vi "IV.vi"(2 "Run uninterrupted?":bool, 3 "Device Category IN:":string(combo)="R0" caption="Device Category:", 4 "Batch No.:":string, 5 "Wafer Serial No.:":string, 6 "Sensor Serial No.:":string) -> (0 "Done!":bool)   [LabVIEW 2018]
doc: "Performs IV measurements according to ATLAS ITk Quality Control Specifications."
uses:
  general_VIs/globals/QC_MeasurementSetup.vi
  general_VIs/globals/QC_RunInformation.vi
  InstrControl/InstrumentSetup.vi
  InstrControl/Switching/Switching.lvclass
  InstrControl/SupplyControl/SupplyControl.lvclass
  InstrControl/ArduinoControl/ArduinoControl.lvclass
  <vilib>/Analysis/NI_AALBase.lvlib
  InstrControl/InstrControl.lvclass
panel:
  out "Initial volts [V]":dbl format="%.1f"
  out "Final volts [V]":dbl=-700.0 format="%.1f"
  out "step [V]":dbl=10.0 format="%.1f"
  out "step interval [s]":i32=10
  out "Volts":dbl[](array[numeric]) caption="Volts [V]"
  out "Current":dbl[](array[numeric]) caption="Current [nA]"
  out "Temp.":dbl[](array[numeric]) caption="Temp. [°C]" format="%#.2f"
  out "RH":dbl[](array[numeric]) caption="RH [%]" format="%#.2f"
  out "Igraph":cluster{dbl[], dbl[]}(graph)
  in  "Scales":T1(ring)=enum."Lin - Log"
  in  "Iscale":enum16{"nanoAmps", "microAmps", "milliAmps"}(ring)
  out "positive ramp?":bool
  out "Tab Control":enum32{"IV Setup", "IV Scan"}(tab)
  in  "Switching":string(combo)="LXIPXI Switching"
  in  "User:":string(combo)="Graham"
  in  "IV Supply":string(combo)="Keithley 2410"
  in  "Configurations":bool
  in  "Set current limit?":bool
  in  "Current Limit [µA]":dbl=10.0 min=0.0001 format="%.3f"
  in  "Manufacturer:":string(combo)="Hamamatsu"
  in  "Quit":bool
  in  "Continue":bool
  in  "Temperature":enum16{"Read Arduino", "Enter manually"}(ring)
  in  "abort":bool
  out "Device Category:":string
  out "Batch:":string
  out "Current Volts:":dbl format="%.2f"
  in  "quit (no save)":bool
  in  "Quit & Save":bool
  out "Bias On/Off:":bool
  out "STATUS 1":string
  out "Initiated:":string
  out "Sensor No.:":string
  out "No of steps":u32
  out "Current reading No.":u32
  out "Last reading at:":string
  in  "hold steps":i32
  # "University of\nCambridge"
  # "Strip Sensor QC: IV"
  # "IV Scan parameters:"
  # "Last 5 readings:"
  # "n-4"
  # "n-3"
  # "n-2"
  # "n-1"
  # "n"
  # "Vertical Scale:"
  # "DUT & Test Description"
  # "Hardware"
  # "DUT & Test Description:"
  # "Current status:"
  # "Rdg No:"
  # "out of"
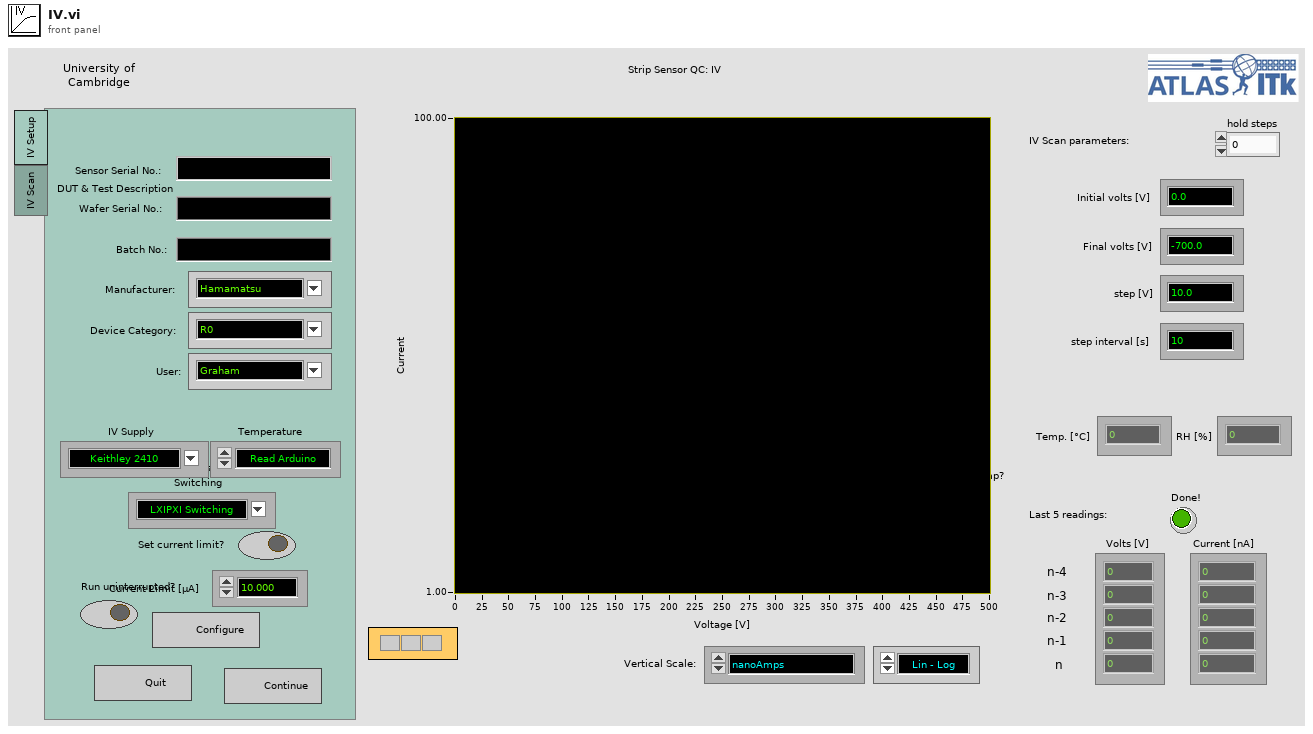
[diagram p1: front panel]
types:
  T1 = enum16{"Lin - Lin", "Log - Lin", "Lin - Log", "Log - log"}
  T2 = enum32{"IV", "CV", "Stability", "Striptest", "Cis", "Ris", "PTP"}
  T3 = enum16{"Reset", "Read Array", "Read Element", "Write Element", "Write Array", "Add Element", "Add Array"}
  T4 = enum16{"Reset", "Ground", "Striptest SMU", "Striptest LCR", "IV", "CV", "Interstrip Cap", "Interstrip Res"}
  T5 = cluster{"Sensor Serial No.:":string, "Wafer Serial No.:":string, "Batch:":string, "Manufacturer:":string, "Device Category:":string, "Database Serial No.:":string, "Initiated:":string, "Test":string, "Instruments used:":string, "Probeplan used:":string, "End of Run comment:":string, "User:":string}
  T6 = cluster{"Institute":string, "Manufacturers":string[], "Devices":string[], "Serialnumbers Lookup DB":string, "Data directory":string, "Backup & screenshot directory":string, "List of known users":string[]}
  T7 = cluster{"Supply":refnum<class "SupplyControl.lvclass">, "Initial Voltage [V]":dbl, "Final Voltage [V]":dbl, "Step Size [V]":dbl, "Step Interval [s]":i32, "Number Of Steps":u32, "Ramp down steps [V]":dbl, "Ramp down Interval [s]":i32, "Set Current Limit?":bool, "Current Limit [µA]":dbl, "Temperature Readout":enum16{"Read Arduino", "Enter manually"}, "Arduino":refnum<class "ArduinoControl.lvclass">, "Supply Name":string, "V_breakdown Limit [V]":dbl, "Switching":refnum<class "Switching.lvclass">}
  T8 = cluster{"VISA address":refnum<visa-resource-name>, "T sensor":enum16{"SHT", "DS"}, "Arduino":refnum<class "ArduinoControl.lvclass">}
  T9 = cluster{"Matrix address":string, "Mux1 address":string, "Mux2 address":string, "Matrix used?":bool, "Switching":refnum<class "Switching.lvclass">, "Matrix X Channels":cluster{"Bias Supply / SMU LO":i32, "Bias Supply / SMU HI":i32, "CV Box LO":i32, "CV Box HI":i32, "CV Box LO IN":i32, "CV Box HI IN":i32, "Volt meter LO":i32, "Volt meter HI":i32, "Mux1 C1":i32, "Mux1 C2":i32, "Mux2 C1":i32, "Mux2 C2":i32}}
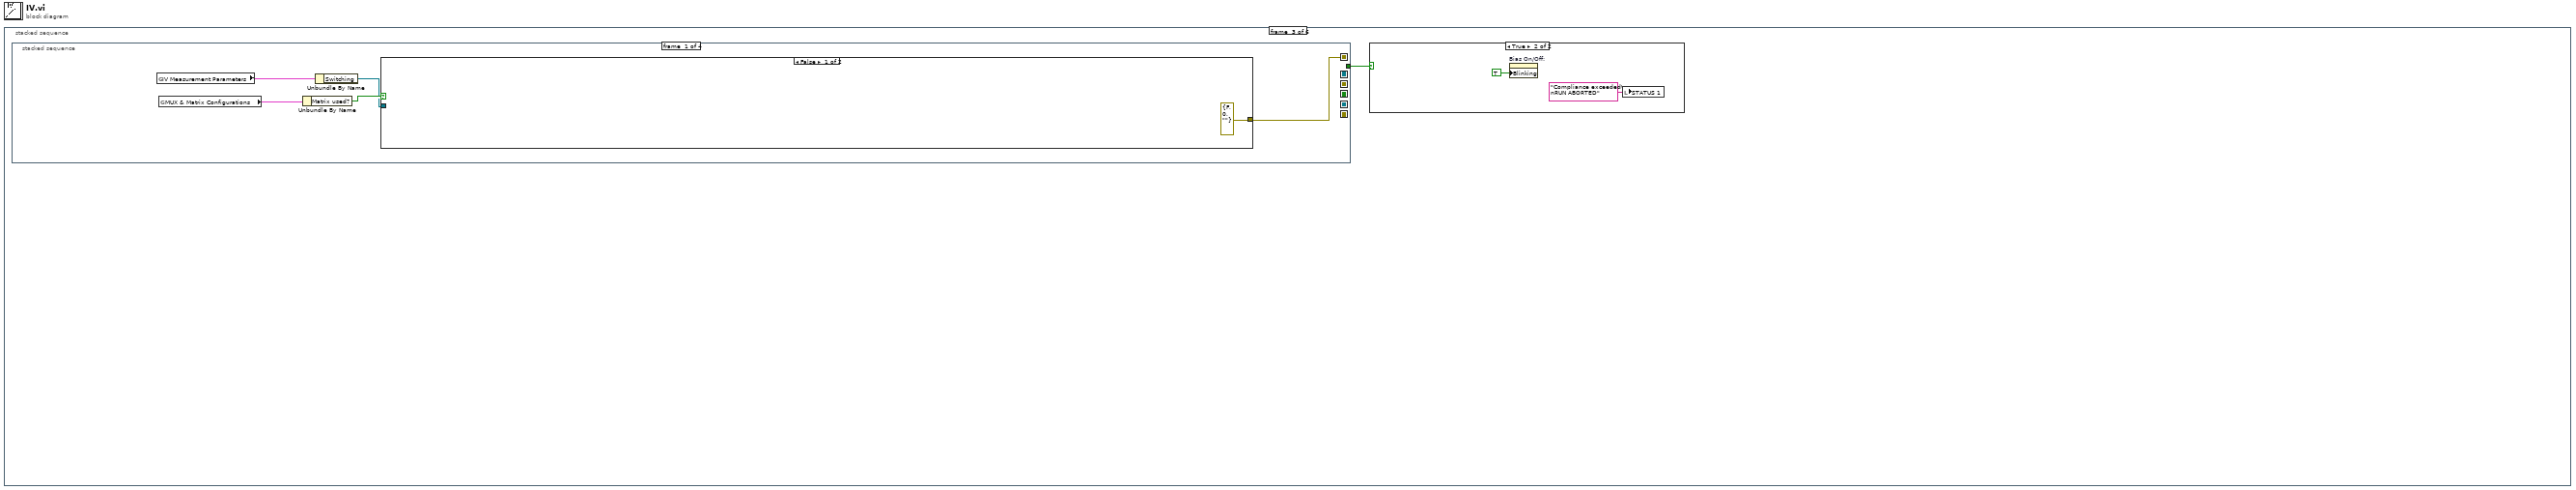
[diagram p0: block diagram]
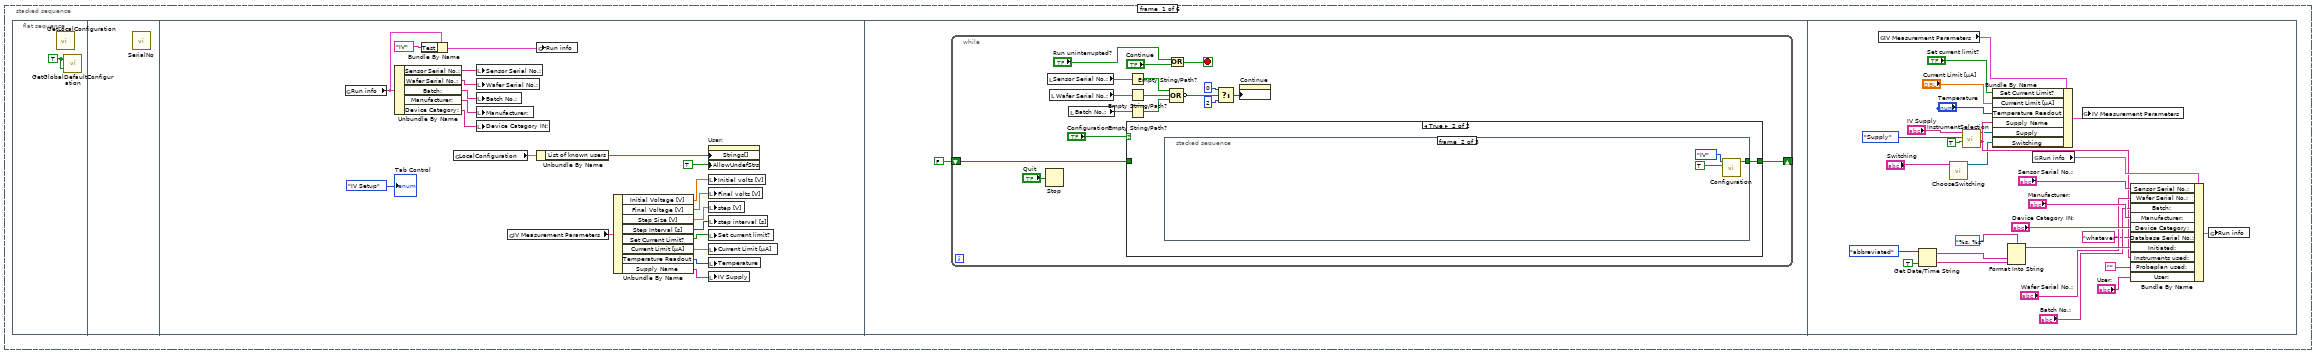
[diagram p2: hidden frame]
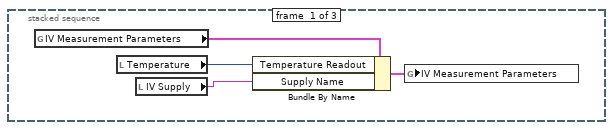
[diagram p4: hidden frame]
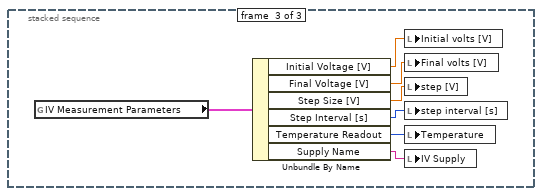
[diagram p5: hidden frame]
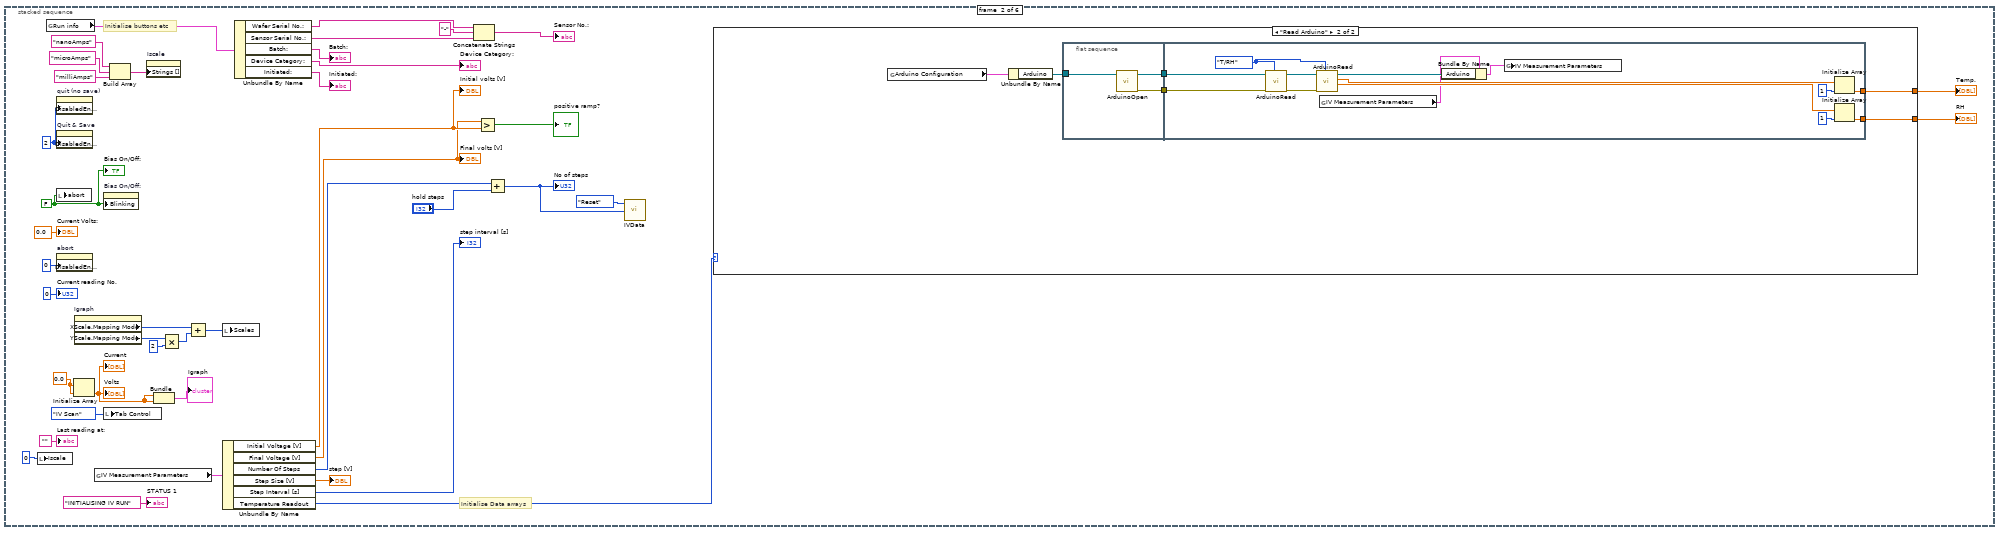
[diagram p6: hidden frame]
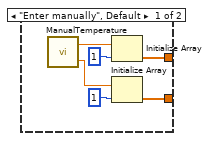
[diagram p7: hidden frame]
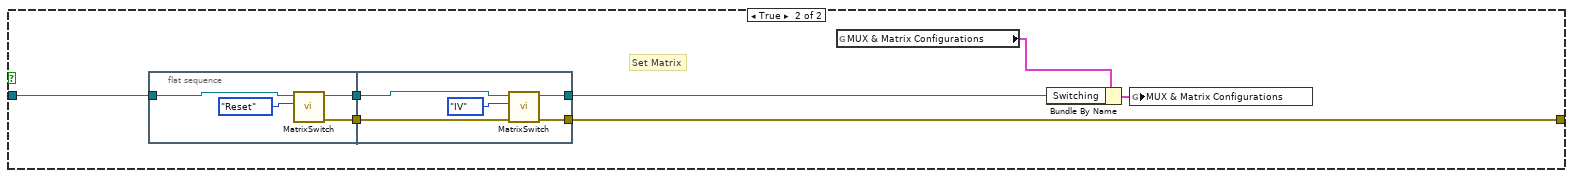
[diagram p8: hidden frame]
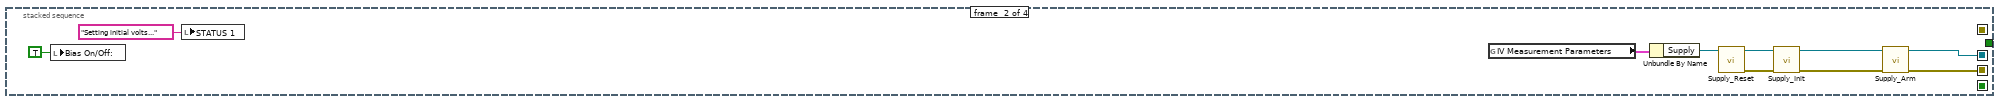
[diagram p9: hidden frame]
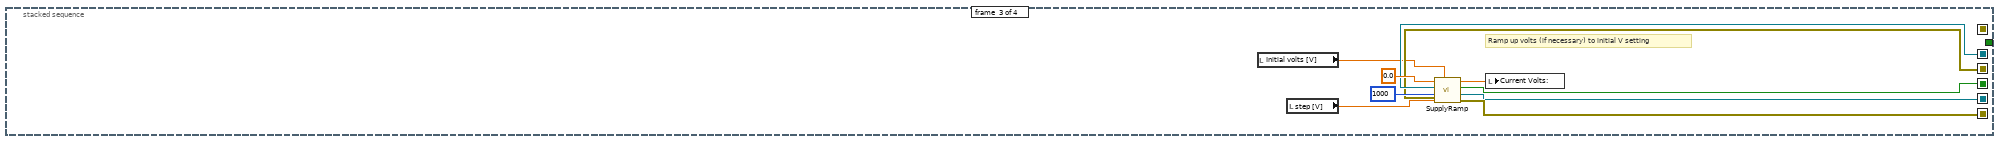
[diagram p10: hidden frame]
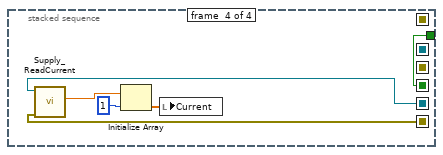
[diagram p11: hidden frame]
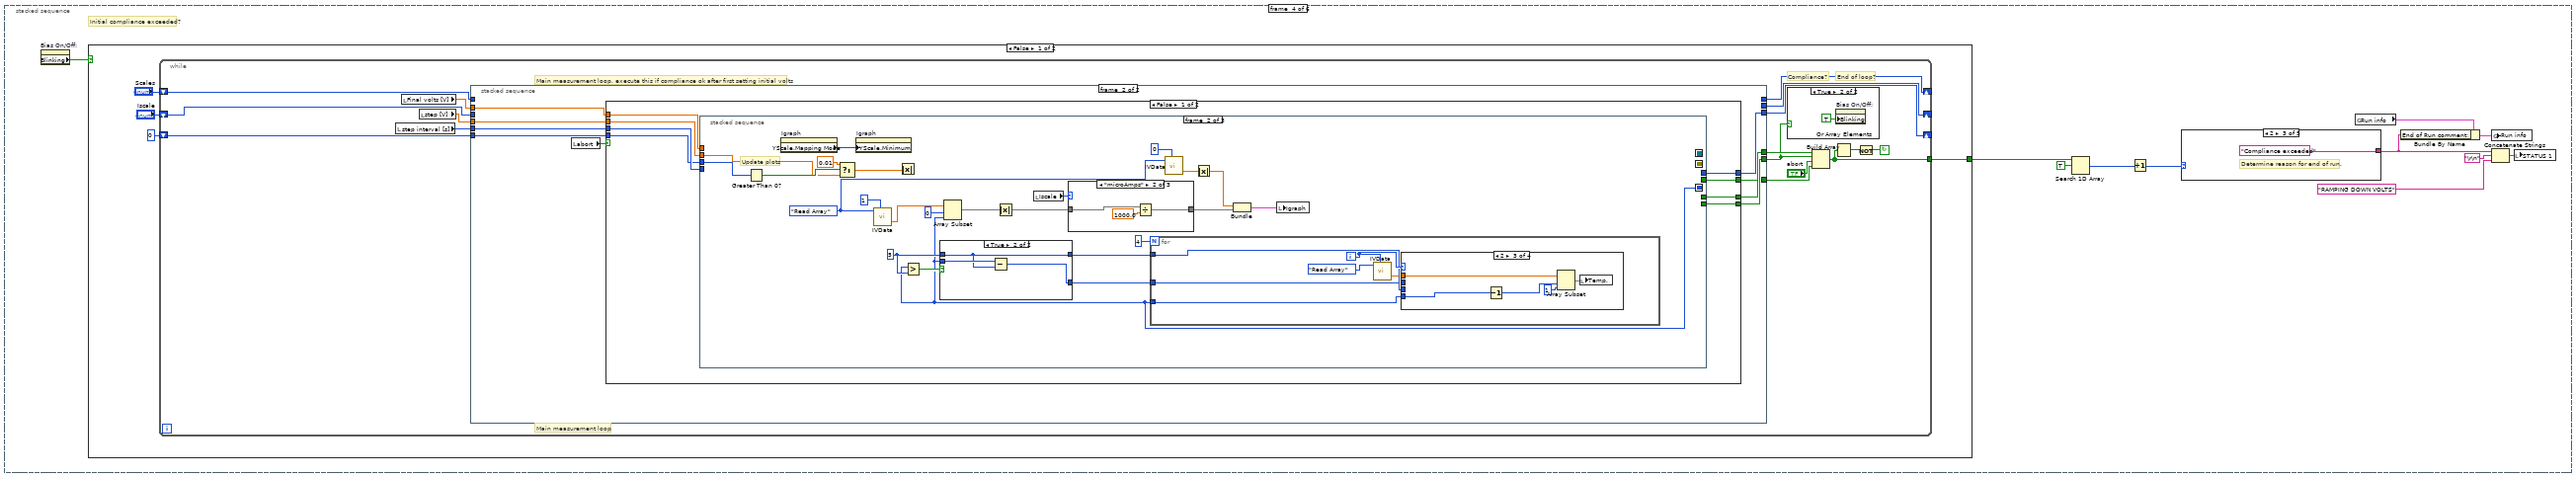
[diagram p13: hidden frame]
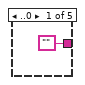
[diagram p14: hidden frame]
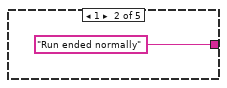
[diagram p15: hidden frame]
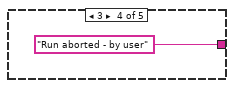
[diagram p16: hidden frame]
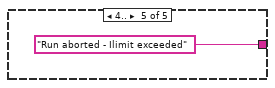
[diagram p17: hidden frame]
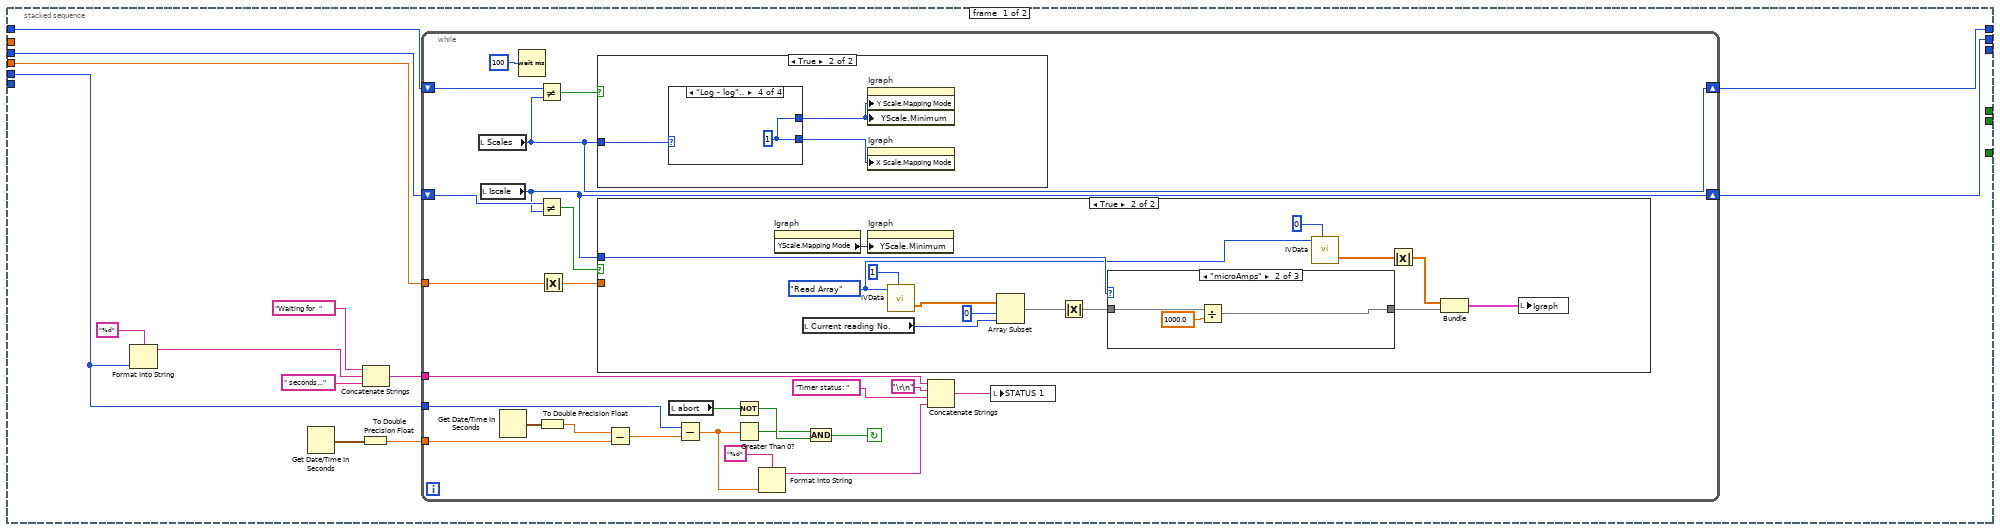
[diagram p18: hidden frame]
diagram:
  n1 = stacked-sequence {
    frame #0 {
      n2 = flat-sequence {
        frame #0 {
          w1 = TRUE
          n3 = call "GetLocalConfiguration.vi"() -> ()  [unwired: 3 in, 1 out]
          n4 = call "GetGlobalDefaultConfiguration.vi"("DO NOT override instruments"=w1, "Read defaults?"=w1) -> ()  [unwired: 1 in, 1 out]
        }
        frame #1 {
          n5 = call "SerialNo.vi"() -> ()  [unwired: 5 in, 1 out]
        }
        frame #2 {
          n6 = global read "QC_RunInformation.vi" "Run info"() -> (w7:T5)
          n7 = Unbundle By Name(w7) -> ("Sensor Serial No.:"=w6:string, "Wafer Serial No.:"=w5:string, "Batch:"=w4:string, "Manufacturer:"=w3:string, "Device Category:"=w2:string)
          n8 = Bundle By Name(cluster=w7, "Test"="IV") -> (w13:T5)
          n9 = global read "QC_RunInformation.vi" "LocalConfiguration"() -> (w16:T6)
          n10 = local write "Sensor Serial No.:"(w6) -> ()
          n11 = local write "Wafer Serial No.:"(w5) -> ()
          n12 = local write "Batch No.:"(w4) -> ()
          n13 = local write "Manufacturer:"(w3) -> ()
          n14 = local write "Device Category IN:"(w2) -> ()
          n15 = global read "QC_MeasurementSetup.vi" "IV Measurement Parameters"() -> (w19:T7)
          n16 = global write "QC_RunInformation.vi" "Run info"(w13) -> ()
          n17 = Unbundle By Name(w16) -> ("List of known users"=w15:string[])
          n18 = Unbundle By Name(w19) -> ("Initial Voltage [V]"=w11:dbl, "Final Voltage [V]"=w10:dbl, "Step Size [V]"=w9:dbl, "Step Interval [s]"=w8:i32, "Set Current Limit?"=w18:bool, "Current Limit [µA]"=w17:dbl, "Temperature Readout"=w21:enum16{"Read Arduino", "Enter manually"}, "Supply Name"=w20:string)
          n19 = property on="User:" class="CmbBox"("Strings[]"=w15, "AllowUndefStrs"=TRUE) -> ()  [unwired: 2 in, 2 out]
          n20 = local write "Initial volts [V]"(w11) -> ()
          n21 = local write "Final volts [V]"(w10) -> ()
          n22 = local write "step [V]"(w9) -> ()
          n23 = local write "step interval [s]"(w8) -> ()
          n24 = local write "Set current limit?"(w18) -> ()
          n25 = local write "Current Limit [µA]"(w17) -> ()
          n26 = local write "Temperature"(w21) -> ()
          n27 = local write "IV Supply"(w20) -> ()
          "Tab Control" <- enum32{"IV Setup", "IV Scan"}."IV Setup" ("Tab Control")
        }
        frame #3 {
          n28 = while {
            shift-right: [w28] -> _
            shift-left: FALSE -> [w27]
            stop <- w24 stop-if-true
            n29 = Stop(stop? (T)="Quit") -> ()
            n30 = local read "Sensor Serial No.:"() -> (w39:string)
            n31 = local read "Wafer Serial No.:"() -> (w38:string)
            n32 = local read "Batch No.:"() -> (w30:string)
            n33 = case shown="True" "Configurations" {
              tunnel: [w41 w42] -> w28
              tunnel: w27 -> [w41 _]
              frame False {
              }
              frame True {
                n34 = stacked-sequence {
                  tunnel: [_ w47 _] -> w42
                  frame #0 {
                    n35 = global read "QC_MeasurementSetup.vi" "IV Measurement Parameters"() -> (w43:T7)
                    n36 = local read "Temperature"() -> (w44:enum16{"Read Arduino", "Enter manually"})
                    n37 = local read "IV Supply"() -> (w45:string)
                    n38 = Bundle By Name(cluster=w43, "Temperature Readout"=w44, "Supply Name"=w45) -> (w46:T7)
                    n39 = global write "QC_MeasurementSetup.vi" "IV Measurement Parameters"(w46) -> ()
                  }
                  frame #1 {
                    n40 = call "Configuration.vi"("Open from\nscan VI"=TRUE, "Measurements"=T2."IV") -> ("configured?"=w47:bool)  [unwired: 9 in]
                  }
                  frame #2 {
                    n41 = global read "QC_MeasurementSetup.vi" "IV Measurement Parameters"() -> (w54:T7)
                    n42 = Unbundle By Name(w54) -> ("Initial Voltage [V]"=w53:dbl, "Final Voltage [V]"=w52:dbl, "Step Size [V]"=w51:dbl, "Step Interval [s]"=w50:i32, "Temperature Readout"=w55:enum16{"Read Arduino", "Enter manually"}, "Supply Name"=w56:string)
                    n43 = local write "Initial volts [V]"(w53) -> ()
                    n44 = local write "Final volts [V]"(w52) -> ()
                    n45 = local write "step [V]"(w51) -> ()
                    n46 = local write "step interval [s]"(w50) -> ()
                    n47 = local write "Temperature"(w55) -> ()
                    n48 = local write "IV Supply"(w56) -> ()
                  }
                }
              }
            }
            n49 = Empty String/Path?(string/path=w39) -> (empty?=w36:bool)
            n50 = Empty String/Path?(string/path=w38) -> (empty?=w37:bool)
            n51 = Empty String/Path?(string/path=w30) -> (empty?=w29:bool)
            n52 = Or(x="Run uninterrupted?", y="Continue") -> (x .or. y?=w24:bool)
            n53 = Compound Arithmetic op=OR(w36, w37, w29) -> (invert w35:bool)
            n54 = Select(t=0, s=w35, f=2) -> (s? t:f=w32:i32)
            n55 = property on="Continue" class="Bool"("DisabledEnum"=w32) -> ()  [unwired: 2 in, 2 out]
          }
        }
        frame #4 {
          n56 = global read "QC_MeasurementSetup.vi" "IV Measurement Parameters"() -> (w83:T7)
          n57 = Get Date/Time String(date format (0)=enum16{"short", "long", "abbreviated"}."abbreviated", want seconds? (F)=TRUE) -> (date string=w78:string, time string=w77:string)  [unwired: 1 in]
          n58 = call "ChooseSwitching.vi"("Instrument name IN"="Switching") -> ("Switching.lvclass"=w57:refnum<class "Switching.lvclass">)  [unwired: 9 in, 1 out]
          n59 = call "InstrumentSelection.vi"("Verify GPIB address"=TRUE, "Instrument type"=enum16{"Supply", "LCR", "Multimeter"}."Supply", "Instrument name IN"="IV Supply") -> ("Instrument name OUT"=w61:string, "Supply"=w60:refnum<class "SupplyControl.lvclass">)  [unwired: 4 in, 3 out]
          n60 = Bundle By Name(cluster=w83, "Set Current Limit?"="Set current limit?", "Current Limit [µA]"="Current Limit [µA]", "Temperature Readout"="Temperature", "Supply Name"=w61, "Supply"=w60, "Switching"=w57) -> (w84:T7)
          n61 = Format Into String(format string="%s, %s", w78, w77) -> (resulting string=w73:string)  [unwired: 2 in, 1 out]
          n62 = global read "QC_RunInformation.vi" "Run info"() -> (w75:T5)
          n63 = global write "QC_MeasurementSetup.vi" "IV Measurement Parameters"(w84) -> ()
          n64 = Bundle By Name(cluster=w75, "Sensor Serial No.:"="Sensor Serial No.:", "Wafer Serial No.:"="Wafer Serial No.:", "Batch:"="Batch No.:", "Manufacturer:"="Manufacturer:", "Device Category:"="Device Category IN:", "Database Serial No.:"="whatever", "Initiated:"=w73, "Instruments used:"=w61, "Probeplan used:"="", "User:"="User:") -> (w74:T5)
          n65 = global write "QC_RunInformation.vi" "Run info"(w74) -> ()
        }
      }
    }
    frame #1 {
      w109 = 2
      w116 = 0.0
      w108 = FALSE ("Visible")
      # "Initialise buttons etc"
      # "Initialise Data arrays"
      n66 = local write "Iscale"(u16 0 ("Scale")) -> ()
      n67 = global read "QC_RunInformation.vi" "Run info"() -> (w125:T5)
      n68 = property on="quit (no save)" class="Bool"("DisabledEnum"=w109) -> ()  [unwired: 2 in, 2 out]
      n69 = property on="Quit & Save" class="Bool"("DisabledEnum"=w109) -> ()  [unwired: 2 in, 2 out]
      n70 = local write "abort"(w108) -> ()
      n71 = property on="abort" class="Bool (strict)"("DisabledEnum"=0) -> ()  [unwired: 2 in, 2 out]
      n72 = Initialize Array(w116, w116) -> (w85:dbl[])
      "Volts" <- w85
      "Current" <- w85
      n73 = property on="Igraph" class="XYGraph (strict)"() -> ("XScale.Mapping Mode"=w101:u8, "YScale.Mapping Mode"=w100:u8)  [unwired: 2 in, 2 out]
      n74 = global read "QC_MeasurementSetup.vi" "IV Measurement Parameters"() -> (w97:T7)
      n75 = property on="Bias On/Off:" class="Bool (strict)"("Blinking"=w108) -> ()  [unwired: 2 in, 2 out]
      n76 = local write "Tab Control"(enum32{"IV Setup", "IV Scan"}."IV Scan" ("Tab Control")) -> ()
      n77 = Build Array("nanoAmps", "microAmps", "milliAmps") -> (w122:string[])
      n78 = property on="Iscale" class="Enum (strict)"("Strings []"=w122) -> ()  [unwired: 2 in, 2 out]
      n79 = Bundle(w85, w85) -> (→"Igraph":cluster{dbl[], dbl[]})  [unwired: 1 in]
      n80 = Multiply(x=w100, y=2) -> (x*y=w103:i32)
      n81 = Add(x=w101, y=w103) -> (x+y=w99:i32)
      n82 = local write "Scales"(w99) -> ()
      n83 = Unbundle By Name(w97) -> ("Initial Voltage [V]"=w107:dbl, "Final Voltage [V]"=w106:dbl, "Number Of Steps"=w88:u32, "Step Size [V]"=→"step [V]":dbl, "Step Interval [s]"=→"step interval [s]":i32, "Temperature Readout"=w110:enum16{"Read Arduino", "Enter manually"})
      "Initial volts [V]" <- w107
      "Final volts [V]" <- w106
      n84 = Unbundle By Name(w125) -> ("Wafer Serial No.:"=w94:string, "Sensor Serial No.:"=w93:string, "Batch:"=→"Batch:":string, "Device Category:"=→"Device Category:":string, "Initiated:"=→"Initiated:":string)
      n85 = Concatenate Strings(w94, "-", w93) -> (→"Sensor No.:":string)
      n86 = Greater?(x=w106, y=w107) -> (0:→"positive ramp?":bool)
      n87 = Add(x=w88, y="hold steps") -> (x+y=w87:u32)
      "No of steps" <- w87
      n88 = call "IVData.vi"("Action"=T3."Reset", "Array Size / Index"=w87) -> ()  [unwired: 3 in, 2 out]
      n89 = case shown="\"Read Arduino\"" w110 {
        tunnel: [w131 w138] -> w113
        tunnel: [w128 w137] -> w98
        frame "Enter manually", Default {
          n90 = call "ManualTemperature.vi"() -> ("Humidity [%] out"=w127:dbl, "Temperature [°C] out"=w132:dbl)
          n91 = Initialize Array(w132, 1) -> (w131:dbl[])
          n92 = Initialize Array(w127, 1) -> (w128:dbl[])
        }
        frame "Read Arduino" {
          n93 = global read "InstrumentSetup.vi" "Arduino Configuration"() -> (w134:T8)
          n94 = Unbundle By Name(w134) -> ("Arduino"=w133:refnum<class "ArduinoControl.lvclass">)
          n95 = flat-sequence {
            tunnel: [w139] -> w136
            tunnel: [w141] -> w135
            tunnel: w133 -> [w140]
            tunnel: [w155] -> w138
            tunnel: [w152] -> w137
            tunnel: w136 -> [w146]
            tunnel: w135 -> [w145]
            frame #0 {
              n96 = call "ArduinoOpen.vi"("ArduinoControl in"=w140) -> ("error out"=w141:errorcluster, "ArduinoControl out"=w139:refnum<class "ArduinoControl.lvclass">)  [unwired: 9 in]
            }
            frame #1 {
              w142 = enum16{"T/RH", "Interlock", "Edgesense"}."T/RH" ("Arduino function")
              n97 = call "ArduinoRead.vi"("Arduino function"=w142, "error in (no error)"=w145, "ArduinoControl in"=w146) -> ("error out"=w144:errorcluster, "ArduinoControl out"=w143:refnum<class "ArduinoControl.lvclass">)  [unwired: 3 in, 4 out]
              n98 = call "ArduinoRead.vi"("Arduino function"=w142, "error in (no error)"=w144, "ArduinoControl in"=w143) -> ("rel. Humidity [%]"=w150:dbl, "Temperature [°C]"=w151:dbl, "ArduinoControl out"=w149:refnum<class "ArduinoControl.lvclass">)  [unwired: 3 in, 3 out]
              n99 = global read "QC_MeasurementSetup.vi" "IV Measurement Parameters"() -> (w148:T7)
              n100 = Bundle By Name(cluster=w148, "Arduino"=w149) -> (w147:T7)
              n101 = global write "QC_MeasurementSetup.vi" "IV Measurement Parameters"(w147) -> ()
              n102 = Initialize Array(w151, 1) -> (w155:dbl[])
              n103 = Initialize Array(w150, 1) -> (w152:dbl[])
            }
          }
        }
      }
      "Temp." <- w113
      "RH" <- w98
      "STATUS 1" <- "INITIALISING IV RUN"
      "Bias On/Off:" <- w108
      "Last reading at:" <- ""
      "Current reading No." <- u32 0 ("Current reading No.")
      "Current Volts:" <- 0.0 ("Current Volts:")
    }
    frame #2 {
      n104 = stacked-sequence {
        seq-local: [_ w184 _ _] -> [_ _ w193 _]
        seq-local: [_ w183 _ _] -> [_ _ w192 _]
        seq-local: [_ _ w194 _] -> [_ _ _ w202]
        seq-local: [_ _ w191 _] -> [_ _ _ w203]
        seq-local: [_ _ w190 _] -> [_ _ _ w204]
        seq-local: [w159 _ _ _] -> [_ _ _ _]
        tunnel: [_ _ _ w202] -> w156
        frame #0 {
          n105 = global read "QC_MeasurementSetup.vi" "IV Measurement Parameters"() -> (w158:T7)
          n106 = global read "InstrumentSetup.vi" "MUX & Matrix Configurations"() -> (w160:T9)
          n107 = Unbundle By Name(w160) -> ("Matrix used?"=w161:bool)
          n108 = Unbundle By Name(w158) -> ("Switching"=w157:refnum<class "Switching.lvclass">)
          n109 = case shown="False" w161 {
            tunnel: w157 -> [_ w163]
            tunnel: [errorcluster {"status"=FALSE, "code"=0, "source"=""} ("error constant") w164] -> w159
            frame False {
            }
            frame True {
              # "Set Matrix"
              n110 = flat-sequence {
                tunnel: [w173] -> w169
                tunnel: [w172] -> w168
                tunnel: w163 -> [w170]
                tunnel: w169 -> [w178]
                tunnel: w168 -> [w177]
                tunnel: [w176] -> w165
                tunnel: [w175] -> w164
                frame #0 {
                  n111 = call-dynamic "MatrixSwitch.vi"("Action"=T4."Reset", "Switching in"=w170) -> ("error out"=w173:errorcluster, "Switching out"=w172:refnum<class "Switching.lvclass">)  [unwired: 8 in]
                }
                frame #1 {
                  n112 = call-dynamic "MatrixSwitch.vi"("error in (no error)"=w178, "Action"=T4."IV", "Switching in"=w177) -> ("error out"=w175:errorcluster, "Switching out"=w176:refnum<class "Switching.lvclass">)  [unwired: 7 in]
                }
              }
              n113 = global read "InstrumentSetup.vi" "MUX & Matrix Configurations"() -> (w166:T9)
              n114 = Bundle By Name(cluster=w166, "Switching"=w165) -> (w167:T9)
              n115 = global write "InstrumentSetup.vi" "MUX & Matrix Configurations"(w167) -> ()
            }
          }
        }
        frame #1 {
          n116 = local write "Bias On/Off:"(TRUE ("Compliance?")) -> ()
          n117 = local write "STATUS 1"("Setting initial volts..." ("STATUS 1")) -> ()
          n118 = global read "QC_MeasurementSetup.vi" "IV Measurement Parameters"() -> (w182:T7)
          n119 = Unbundle By Name(w182) -> ("Supply"=w179:refnum<class "SupplyControl.lvclass">)
          n120 = call-dynamic "Supply_Reset.vi"("SupplyControl in"=w179) -> ("error out"=w186:errorcluster, "SupplyControl out"=w188:refnum<class "SupplyControl.lvclass">)  [unwired: 9 in]
          n121 = call-dynamic "Supply_Init.vi"("error in (no error)"=w186, "SupplyControl in"=w188) -> ("error out"=w185:errorcluster, "SupplyControl out"=w187:refnum<class "SupplyControl.lvclass">)  [unwired: 8 in]
          n122 = call-dynamic "Supply_Arm.vi"("error in (no error)"=w185, "SupplyControl in"=w187) -> ("error out"=w183:errorcluster, "SupplyControl out"=w184:refnum<class "SupplyControl.lvclass">)  [unwired: 8 in]
        }
        frame #2 {
          # "Ramp up volts (if necessary) to initial V setting"
          n123 = local read "Initial volts [V]"() -> (w189:dbl)
          n124 = local read "step [V]"() -> (w195:dbl)
          n125 = call "SupplyRamp.vi"("error in"=w192, "Requested Voltage"=w189, "Step Size"=w195, "Step Delay"=1000, "Supply IN"=w193, "Starting Voltage"=0.0) -> ("error out"=w191:errorcluster, "Supply OUT"=w190:refnum<class "SupplyControl.lvclass">, "Compliance exceeded"=w194:bool, "Current Voltage"=w198:dbl)  [unwired: 2 in]
          n126 = local write "Current Volts:"(w198) -> ()
        }
        frame #3 {
          n127 = call-dynamic "Supply_ReadCurrent.vi"("error in (no error)"=w203, "SupplyControl in"=w204) -> ("Current in nA"=w200:dbl)  [unwired: 7 in, 2 out]
          n128 = Initialize Array(w200, 1) -> (w199:dbl[])
          n129 = local write "Current"(w199) -> ()
        }
      }
      n130 = case shown="True" w156 {
        frame False {
        }
        frame True {
          n131 = property on="Bias On/Off:" class="Bool (strict)"("Blinking"=TRUE) -> ()  [unwired: 2 in, 2 out]
          n132 = local write "STATUS 1"("Compliance exceeded\nRUN ABORTED") -> ()
        }
      }
    }
    frame #3 {
      # "Initial compliance exceeded?"
      n133 = property on="Bias On/Off:" class="Bool (strict)"() -> ("Blinking"=w217:bool)  [unwired: 2 in, 2 out]
      n134 = case shown="False" w217 {
        tunnel: [w226 w476] -> w216
        frame False {
          n135 = while {
            shift-left: "Iscale" -> [w238]
            shift-right: [w237] -> _
            shift-left: "Scales" -> [w239]
            shift-right: [w240] -> _
            tunnel: [w236] -> w226
            shift-right: [w227] -> _
            shift-left: 0 -> [w228]
            stop <- w241 continue-if-true
            # "Main measurement loop"
            # "End of loop?"
            # "Compliance?"
            # "Main measurement loop. execute this if compliance ok after first setting initial volts"
            n136 = local read "step interval [s]"() -> (w233:i32)
            n137 = local read "Final volts [V]"() -> (w234:dbl)
            n138 = local read "step [V]"() -> (w235:dbl)
            n139 = stacked-sequence {
              tunnel: [w255 _] -> w240
              tunnel: w235 -> [w252 w319]
              tunnel: [_ w318] -> w230
              tunnel: w234 -> [_ w317]
              tunnel: w233 -> [w243 w316]
              tunnel: [_ w315] -> w232
              tunnel: w239 -> [w254 _]
              tunnel: w238 -> [w253 _]
              tunnel: [w251 _] -> w237
              tunnel: [_ w313] -> w231
              tunnel: w228 -> [_ w312]
              tunnel: [_ w311] -> w227
              frame #0 {
                n140 = Format Into String(format string="%d", w243) -> (resulting string=w248:string)  [unwired: 2 in, 1 out]
                n141 = Get Date/Time In Seconds() -> (seconds since 1Jan1904=w245:timestamp)
                n142 = To Double Precision Float(number=w245) -> (double precision float=w246:dbl)
                n143 = Concatenate Strings("Waiting for  ", w248, " seconds...") -> (w244:string)
                n144 = while {
                  tunnel: w252 -> [w264]
                  shift-left: w253 -> [w268]
                  shift-right: [w261] -> w251
                  shift-left: w254 -> [w269]
                  shift-right: [w270] -> w255
                  tunnel: w244 -> [w262]
                  tunnel: w243 -> [w274]
                  tunnel: w246 -> [w275]
                  stop <- w276 continue-if-true
                  n145 = local read "Scales"() -> (w270:T1)
                  n146 = local read "Iscale"() -> (w261:enum16{"nanoAmps", "microAmps", "milliAmps"})
                  n147 = Get Date/Time In Seconds() -> (seconds since 1Jan1904=w260:timestamp)
                  n148 = Wait (ms)(milliseconds to wait=u32 100) -> ()  [unwired: 1 out]
                  n149 = Not Equal?(x=w269, y=w270) -> (x != y?=w271:bool)
                  n150 = Not Equal?(x=w268, y=w261) -> (x != y?=w259:bool)
                  n151 = To Double Precision Float(number=w260) -> (double precision float=w280:dbl)
                  n152 = Absolute Value(x=w264) -> (abs(x)=w263:dbl)
                  n153 = case shown="True" w271 {
                    tunnel: w270 -> [_ w304]
                    frame False {
                    }
                    frame True {
                      n154 = case shown="\"Log - log\".." w304 {
                        tunnel: [w305 1 0 w310] -> w303
                        tunnel: [w305 0 1 w310] -> w302
                        frame .."Lin - Lin" {
                          w305 = 0
                        }
                        frame "Log - Lin" {
                        }
                        frame "Lin - Log" {
                        }
                        frame "Log - log".. {
                          w310 = 1
                        }
                      }
                      n155 = property on="Igraph" class="XYGraph (strict)"("Y Scale.Mapping Mode"=w302, "YScale.Minimum"=w302) -> ()  [unwired: 2 in, 2 out]
                      n156 = property on="Igraph" class="XYGraph (strict)"("X Scale.Mapping Mode"=w303) -> ()  [unwired: 2 in, 2 out]
                    }
                  }
                  n157 = case shown="True" w259 {
                    tunnel: w263 -> [_ _]
                    tunnel: w261 -> [_ w289]
                    frame False {
                    }
                    frame True {
                      w283 = T3."Read Array" ("Action")
                      n158 = property on="Igraph" class="XYGraph (strict)"() -> ("YScale.Mapping Mode"=w285:u8)  [unwired: 2 in, 2 out]
                      n159 = local read "Current reading No."() -> (w291:u32)
                      n160 = property on="Igraph" class="XYGraph (strict)"("YScale.Minimum"=w285) -> ()  [unwired: 2 in, 2 out]
                      n161 = call "IVData.vi"("Action"=w283, "Array No."=u32 1 ("Action")) -> ("Array OUT"=w292:dbl[])  [unwired: 3 in, 1 out]
                      n162 = Array Subset(array=w292, index=0, length=w291) -> (w288:dbl[])
                      n163 = Absolute Value(x=w288) -> (abs(x)=w287:dbl[])
                      n164 = case shown="\"microAmps\"" w289 {
                        tunnel: [w295 w296 w300] -> w294
                        tunnel: w287 -> [w295 w298 w301]
                        frame .."nanoAmps" {
                        }
                        frame "microAmps" {
                          n165 = Divide(x=w298, y=1000.0) -> (x/y=w296:dbl[])
                        }
                        frame "milliAmps".. {
                          n166 = Divide(x=w301, y=1000000.0) -> (x/y=w300:dbl[])
                        }
                      }
                      n167 = call "IVData.vi"("Action"=w283, "Array No."=u32 0 ("Action")) -> ("Array OUT"=w282:dbl[])  [unwired: 3 in, 1 out]
                      n168 = Absolute Value(x=w282) -> (abs(x)=w281:dbl[])
                      n169 = Bundle(w281, w294) -> (w290:cluster{dbl[], dbl[]})  [unwired: 1 in]
                      n170 = local write "Igraph"(w290) -> ()
                    }
                  }
                  n171 = Subtract(x=w280, y=w275) -> (x-y=w257:dbl)
                  n172 = local read "abort"() -> (w273:bool)
                  n173 = Subtract(x=w274, y=w257) -> (x-y=w256:dbl)
                  n174 = Not(x=w273) -> (.not. x?=w279:bool)
                  n175 = Greater Than 0?(x=w256) -> (x > 0?=w258:bool)
                  n176 = Format Into String(format string="%d", w256) -> (resulting string=w278:string)  [unwired: 2 in, 1 out]
                  n177 = And(x=w258, y=w279) -> (x .and. y?=w276:bool)
                  n178 = Concatenate Strings(w262, "\r\n", "Timer status: ", w278) -> (w272:string)
                  n179 = local write "STATUS 1"(w272) -> ()
                }
              }
              frame #1 {
                n180 = local read "abort"() -> (w314:bool)
                n181 = case shown="False" w314 {
                  tunnel: [w327 w473] -> w315
                  tunnel: w316 -> [w326 _]
                  tunnel: w317 -> [w325 _]
                  tunnel: [w323 w473] -> w318
                  tunnel: w319 -> [w324 _]
                  tunnel: [w322 w473] -> w313
                  tunnel: w312 -> [w321 w472]
                  tunnel: [w320 w472] -> w311
                  frame False {
                    n182 = stacked-sequence {
                      seq-local: [w342 _ _] -> [_ w377 _]
                      seq-local: [w337 _ _] -> [_ _ w437]
                      seq-local: [w336 _ _] -> [_ _ w438]
                      tunnel: w324 -> [_ w374 w443]
                      tunnel: w325 -> [_ _ w435]
                      tunnel: [_ _ w441] -> w327
                      tunnel: [_ _ w440] -> w323
                      tunnel: w326 -> [_ _ _]
                      tunnel: [w346 _ _] -> w322
                      tunnel: w321 -> [_ w375 w429]
                      tunnel: [_ _ w428] -> w320
                      frame #0 {
                        w340 = T3."Write Element" ("Action")
                        # "SMU data"
                        n183 = Get Date/Time String(want seconds? (F)=TRUE) -> (time string=w343:string)  [unwired: 2 in, 1 out]
                        n184 = local write "Last reading at:"(w343) -> ()
                        n185 = local write "STATUS 1"("Reading current ..." ("status")) -> ()
                        n186 = global read "QC_MeasurementSetup.vi" "IV Measurement Parameters"() -> (w335:T7)
                        n187 = Unbundle By Name(w335) -> ("Supply"=w329:refnum<class "SupplyControl.lvclass">, "Set Current Limit?"=w334:bool, "Current Limit [µA]"=w331:dbl, "Temperature Readout"=w333:enum16{"Read Arduino", "Enter manually"}, "Arduino"=w328:refnum<class "ArduinoControl.lvclass">)
                        n188 = local read "Current reading No."() -> (w339:u32)
                        n189 = case shown="\"Read Arduino\"" w333 {
                          tunnel: [w356 w362] -> w344
                          tunnel: [w353 w361] -> w338
                          tunnel: w328 -> [_ w360]
                          frame "Enter manually", Default {
                            n190 = local read "Temp."() -> (w358:dbl[])
                            n191 = local read "RH"() -> (w354:dbl[])
                            n192 = Index Array(array=w354, index=0) -> (element=w353:dbl)
                            n193 = Index Array(array=w358, index=0) -> (element=w356:dbl)
                          }
                          frame "Read Arduino" {
                            n194 = call "ArduinoRead.vi"("Arduino function"=enum16{"T/RH", "Interlock", "Edgesense"}."T/RH", "ArduinoControl in"=w360) -> ("rel. Humidity [%]"=w361:dbl, "Temperature [°C]"=w362:dbl)  [unwired: 4 in, 4 out]
                          }
                        }
                        n195 = local read "Current Volts:"() -> (w348:dbl)
                        n196 = Multiply(x=w331, y=1000.0) -> (x*y=w330:dbl)
                        n197 = call-dynamic "Supply_ReadCurrent.vi"("SupplyControl in"=w329) -> ("error out"=w336:errorcluster, "Current in nA"=w347:dbl, "SupplyControl out"=w337:refnum<class "SupplyControl.lvclass">)  [unwired: 8 in]
                        n198 = case shown="True" w334 {
                          tunnel: w347 -> [_ w367]
                          tunnel: w330 -> [_ w365]
                          tunnel: [FALSE w364] -> w346
                          frame False {
                          }
                          frame True {
                            n199 = Absolute Value(x=w367) -> (abs(x)=w366:dbl)
                            n200 = Greater?(x=w366, y=w365) -> (0:w364:bool)
                          }
                        }
                        n201 = call "IVData.vi"("Action"=w340, "Array No."=u32 1, "Array Size / Index"=w339, "Data IN"=w347) -> ()  [unwired: 1 in, 2 out]
                        n202 = call "IVData.vi"("Action"=w340, "Array No."=0, "Array Size / Index"=w339, "Data IN"=w348) -> ()  [unwired: 1 in, 2 out]
                        n203 = Increment(x=w339) -> (x+1=w342:u32)
                        n204 = local write "Current reading No."(w342) -> ()
                        n205 = call "IVData.vi"("Action"=w340, "Array No."=u32 2, "Array Size / Index"=w339, "Data IN"=w344) -> ()  [unwired: 1 in, 2 out]
                        n206 = call "IVData.vi"("Action"=w340, "Array No."=u32 3, "Array Size / Index"=w339, "Data IN"=w338) -> ()  [unwired: 1 in, 2 out]
                      }
                      frame #1 {
                        w370 = T3."Read Array" ("Action")
                        w387 = u32 5 ("y")
                        # "Update plots"
                        n207 = Greater Than 0?(x=w375) -> (x > 0?=w376:bool)
                        n208 = property on="Igraph" class="XYGraph (strict)"() -> ("YScale.Mapping Mode"=w378:u8)  [unwired: 2 in, 2 out]
                        n209 = Select(t=0.01, s=w376, f=w374) -> (s? t:f=w373:dbl)
                        n210 = property on="Igraph" class="XYGraph (strict)"("YScale.Minimum"=w378) -> ()  [unwired: 2 in, 2 out]
                        n211 = call "IVData.vi"("Action"=w370, "Array No."=1) -> ("Array OUT"=w389:dbl[])  [unwired: 3 in, 1 out]
                        n212 = Absolute Value(x=w373) -> ()  [unwired: 1 out]
                        n213 = Greater?(x=w377, y=w387) -> (0:w386:bool)
                        n214 = case shown="True" w386 {
                          tunnel: w377 -> [w393 w396]
                          tunnel: w387 -> [_ w395]
                          tunnel: [w393 w395] -> w385
                          tunnel: [0 w394] -> w383
                          frame False {
                          }
                          frame True {
                            n215 = Subtract(x=w396, y=w395) -> (x-y=w394:u32)
                          }
                        }
                        n216 = Array Subset(array=w389, index=0, length=w377) -> (w382:dbl[])
                        n217 = Absolute Value(x=w382) -> (abs(x)=w381:dbl[])
                        n218 = local read "Iscale"() -> (w388:enum16{"nanoAmps", "microAmps", "milliAmps"})
                        n219 = case shown="\"microAmps\"" w388 {
                          tunnel: [w421 w422 w425] -> w391
                          tunnel: w381 -> [w421 w424 w427]
                          frame .."nanoAmps" {
                          }
                          frame "microAmps" {
                            n220 = Divide(x=w424, y=1000.0) -> (x/y=w422:dbl[])
                          }
                          frame "milliAmps".. {
                            n221 = Divide(x=w427, y=1000000.0) -> (x/y=w425:dbl[])
                          }
                        }
                        n222 = for {
                          N: 4 -> [_]
                          tunnel: w385 -> [w401]
                          tunnel: w383 -> [w400]
                          tunnel: w377 -> [w397]
                          i -> [w402]
                          n223 = call "IVData.vi"("Action"=T3."Read Array", "Array No."=w402) -> ("Array OUT"=w399:dbl[])  [unwired: 3 in, 1 out]
                          n224 = case shown="2" w402 {
                            tunnel: w401 -> [w405 w409 _ _]
                            tunnel: w400 -> [w406 w410 _ _]
                            tunnel: w399 -> [w404 w408 w414 w419]
                            tunnel: w397 -> [_ _ w412 w417]
                            frame ..0 {
                              n225 = Array Subset(array=w404, index=w406, length=w405) -> (w403:dbl[])
                              n226 = local write "Volts"(w403) -> ()
                            }
                            frame 1 {
                              n227 = Array Subset(array=w408, index=w410, length=w409) -> (w407:dbl[])
                              n228 = local write "Current"(w407) -> ()
                            }
                            frame 2 {
                              n229 = Decrement(x=w412) -> (x-1=w411:u32)
                              n230 = Array Subset(array=w414, index=w411, length=1) -> (w413:dbl[])
                              n231 = local write "Temp."(w413) -> ()
                            }
                            frame 3.. {
                              n232 = Decrement(x=w417) -> (x-1=w416:u32)
                              n233 = Array Subset(array=w419, index=w416, length=1) -> (w418:dbl[])
                              n234 = local write "RH"(w418) -> ()
                            }
                          }
                        }
                        n235 = call "IVData.vi"("Action"=w370, "Array No."=0) -> ("Array OUT"=w369:dbl[])  [unwired: 3 in, 1 out]
                        n236 = Absolute Value(x=w369) -> (abs(x)=w368:dbl[])
                        n237 = Bundle(w368, w391) -> (w379:cluster{dbl[], dbl[]})  [unwired: 1 in]
                        n238 = local write "Igraph"(w379) -> ()
                      }
                      frame #2 {
                        # "Increment volts and check for end of loop"
                        n239 = local read "positive ramp?"() -> (w439:bool)
                        n240 = local read "Current Volts:"() -> (w430:dbl)
                        n241 = case shown="True" w439 {
                          tunnel: w435 -> [w446 w450]
                          tunnel: w443 -> [w447 w453]
                          tunnel: [w445 w452] -> w431
                          tunnel: [w444 w449] -> w442
                          tunnel: w430 -> [w448 w451]
                          frame False {
                            n242 = Subtract(x=w448, y=w447) -> (x-y=w444:dbl)
                            n243 = Greater Or Equal?(x=w444, y=w446) -> (x >= y?=w445:bool)
                          }
                          frame True {
                            n244 = Add(x=w451, y=w453) -> (x+y=w449:dbl)
                            n245 = Less Or Equal?(x=w449, y=w450) -> (x <= y?=w452:bool)
                          }
                        }
                        n246 = Quotient & Remainder(x=w430, y=w435) -> (x-y*floor(x/y)=w436:dbl, floor(x/y)=w434:dbl)
                        n247 = Not Equal To 0?(x=w436) -> (x != 0?=w432:bool)
                        n248 = Equal To 0?(x=w434) -> (x = 0?=w433:bool)
                        n249 = Or(x=w432, y=w433) -> ()  [unwired: 1 out]
                        n250 = case shown="False" w431 {
                          tunnel: w442 -> [_ w468]
                          tunnel: [w457 FALSE] -> w441
                          tunnel: [FALSE w469] -> w440
                          tunnel: w430 -> [_ w466]
                          tunnel: w438 -> [_ w465]
                          tunnel: w437 -> [_ w464]
                          tunnel: w429 -> [w456 _]
                          tunnel: [w455 0] -> w428
                          frame False {
                            (unwired) TRUE
                            n251 = local read "hold steps"() -> (w454:i32)
                            n252 = Greater Or Equal?(x=w456, y=w454) -> (x >= y?=w457:bool)
                            n253 = Increment(x=w456) -> (x+1=w455:i32)
                          }
                          frame True {
                            n254 = local read "step [V]"() -> (w462:dbl)
                            n255 = local write "STATUS 1"("Incrementing volts.") -> ()
                            n256 = call "SupplyRamp.vi"("error in"=w465, "Requested Voltage"=w468, "Step Size"=w462, "Step Delay"=100, "Supply IN"=w464, "Starting Voltage"=w466) -> ("error out"=w460:errorcluster, "Compliance exceeded"=w469:bool, "Current Voltage"=w463:dbl)  [unwired: 2 in, 1 out]
                            n257 = property on="Bias On/Off:" class="Bool (strict)"("Blinking"=w469) -> ()  [unwired: 2 in, 2 out]
                            n258 = case shown="No Error" w460 {
                              tunnel: w463 -> [w471 _]
                              frame No Error {
                                n259 = local write "Current Volts:"(w471) -> ()
                              }
                              frame Error {
                              }
                            }
                          }
                        }
                      }
                    }
                  }
                  frame True {
                    w473 = FALSE
                  }
                }
              }
            }
            n260 = case shown="True" w230 {
              frame False {
              }
              frame True {
                n261 = property on="Bias On/Off:" class="Bool (strict)"("Blinking"=TRUE) -> ()  [unwired: 2 in, 2 out]
              }
            }
            n262 = Build Array(w232, w230, "abort", w231) -> (w236:bool[])
            n263 = Or Array Elements(Boolean array=w236) -> (logical OR=w242:bool)
            n264 = Not(x=w242) -> (.not. x?=w241:bool)
          }
        }
        frame True {
          w475 = FALSE
          # "compliance was exceeded when first voltage applied."
          # "Flag compliance as reason for end of run"
          n265 = local write "STATUS 1"("Run aborted - compliance exceeded.") -> ()
          n266 = Build Array(w475, TRUE, w475, w475) -> (w476:bool[])
        }
      }
      n267 = Search 1D Array(1D array=w216, element=TRUE) -> (index of element=w214:i32)  [unwired: 1 in]
      n268 = Increment(x=w214) -> (x+1=w213:i32)
      n269 = case shown="2" w213 {
        tunnel: ["" "Run ended normally" "Compliance exceeded" "Run aborted - by user" "Run aborted - Ilimit exceeded"] -> w208
        frame ..0 {
        }
        frame 1 {
        }
        frame 2 {
          # "Determine reason for end of run."
        }
        frame 3 {
        }
        frame 4.. {
        }
      }
      n270 = global read "QC_RunInformation.vi" "Run info"() -> (w212:T5)
      n271 = Bundle By Name(cluster=w212, "End of Run comment:"=w208) -> (w207:T5)
      n272 = global write "QC_RunInformation.vi" "Run info"(w207) -> ()
      n273 = Concatenate Strings(w208, "\r\n", "RAMPING DOWN VOLTS") -> (w211:string)
      n274 = local write "STATUS 1"(w211) -> ()
    }
    frame #4 {
      n275 = stacked-sequence {
        seq-local: [w481 _ _ _ _] -> [_ w492 _ _ _]
        seq-local: [w480 _ _ _ _] -> [_ w491 _ _ _]
        seq-local: [_ w490 _ _ _] -> [_ _ w495 _ _]
        frame #0 {
          # "Ramp down volts now"
          n276 = global read "QC_MeasurementSetup.vi" "IV Measurement Parameters"() -> (w484:T7)
          n277 = Unbundle By Name(w484) -> ("Supply"=w479:refnum<class "SupplyControl.lvclass">, "Ramp down steps [V]"=w483:dbl, "Ramp down Interval [s]"=w482:i32)
          n278 = Multiply(x=w482, y=1000) -> (x*y=w486:i32)
          n279 = local read "Current Volts:"() -> (w489:dbl)
          n280 = call "SupplyRamp.vi"("Requested Voltage"=0.0, "Step Size"=w483, "Step Delay"=w486, "Supply IN"=w479, "Starting Voltage"=w489) -> ("error out"=w481:errorcluster, "Supply OUT"=w480:refnum<class "SupplyControl.lvclass">, "Current Voltage"=w487:dbl)  [unwired: 3 in, 1 out]
          n281 = local write "Current Volts:"(w487) -> ()
        }
        frame #1 {
          # "Tie up loose ends. Set volts to zero and switch to standby"
          n282 = call-dynamic "Supply_Stby.vi"("error in (no error)"=w492, "SupplyControl in"=w491) -> ("error out"=w490:errorcluster)  [unwired: 8 in, 1 out]
        }
        frame #2 {
          n283 = global read "InstrumentSetup.vi" "MUX & Matrix Configurations"() -> (w496:T9)
          n284 = global read "QC_MeasurementSetup.vi" "IV Measurement Parameters"() -> (w494:T7)
          n285 = Unbundle By Name(w496) -> ("Matrix used?"=w497:bool)
          n286 = Unbundle By Name(w494) -> ("Switching"=w493:refnum<class "Switching.lvclass">)
          n287 = case shown="True" w497 {
            tunnel: w493 -> [_ w502]
            tunnel: w495 -> [_ w501]
            frame False {
            }
            frame True {
              n288 = call-dynamic "MatrixSwitch.vi"("error in (no error)"=w501, "Action"=T4."Reset", "Switching in"=w502) -> ("error out"=w498:errorcluster, "Switching out"=w499:refnum<class "Switching.lvclass">)  [unwired: 7 in]
              n289 = call-dynamic "Close.vi"("error in (no error)"=w498, "Switching in"=w499) -> ()  [unwired: 8 in, 2 out]
            }
          }
        }
        frame #3 {
          w507 = 0
          n290 = local write "Bias On/Off:"(FALSE ("Visible")) -> ()
          n291 = local write "Current Volts:"(0.0 ("Current Volts:")) -> ()
          n292 = property on="abort" class="Bool (strict)"("DisabledEnum"=2) -> ()  [unwired: 2 in, 2 out]
          n293 = property on="Quit & Save" class="Bool"("DisabledEnum"=w507) -> ()  [unwired: 2 in, 2 out]
          n294 = property on="quit (no save)" class="Bool"("DisabledEnum"=w507) -> ()  [unwired: 2 in, 2 out]
          n295 = local write "STATUS 1"("Run finished. \nSave data?" ("STATUS 1")) -> ()
        }
        frame #4 {
          n296 = Current VI's Path() -> (path=w509:path)
          n297 = call "SaveJPEG.vi"("Test"="IV", "File Path Control"=w509) -> ()  [unwired: 1 in, 2 out]
        }
      }
    }
    frame #5 {
      # "Loop and await decision on whether to save or junk data"
      n298 = local read "Scales"() -> (w520:T1)
      n299 = local read "Iscale"() -> (w519:enum16{"nanoAmps", "microAmps", "milliAmps"})
      n300 = while {
        shift-left: w519 -> [w566]
        shift-right: [w565] -> _
        shift-left: w520 -> [w568]
        shift-right: [w567] -> _
        tunnel: ["Quit & Save"] -> w522
        tunnel: ["quit (no save)"] -> w521
        stop <- w563 continue-if-true
        n301 = local read "Scales"() -> (w567:T1)
        n302 = local read "Iscale"() -> (w565:enum16{"nanoAmps", "microAmps", "milliAmps"})
        n303 = Not Equal?(x=w568, y=w567) -> (x != y?=w561:bool)
        n304 = Not Equal?(x=w566, y=w565) -> (x != y?=w560:bool)
        n305 = case shown="True" w561 {
          tunnel: w567 -> [_ w595]
          frame False {
          }
          frame True {
            n306 = case shown="..\"Lin - Lin\"" w595 {
              tunnel: [w596 1 0 w601] -> w594
              tunnel: [w596 0 1 w601] -> w593
              frame .."Lin - Lin" {
                w596 = 0
              }
              frame "Log - Lin" {
              }
              frame "Lin - Log" {
              }
              frame "Log - log".. {
                w601 = 1
              }
            }
            n307 = property on="Igraph" class="XYGraph (strict)"("X Scale.Mapping Mode"=w594) -> ()  [unwired: 2 in, 2 out]
            n308 = property on="Igraph" class="XYGraph (strict)"("Y Scale.Mapping Mode"=w593, "YScale.Minimum"=w593) -> ()  [unwired: 2 in, 2 out]
          }
        }
        n309 = case shown="True" w560 {
          tunnel: w565 -> [_ w581]
          frame False {
          }
          frame True {
            w574 = T3."Read Array" ("Action")
            n310 = property on="Igraph" class="XYGraph (strict)"() -> ("YScale.Mapping Mode"=w577:u8)  [unwired: 2 in, 2 out]
            n311 = property on="Igraph" class="XYGraph (strict)"("YScale.Minimum"=w577) -> ()  [unwired: 2 in, 2 out]
            n312 = global read "QC_MeasurementSetup.vi" "IV Measurement Parameters"() -> (w576:T7)
            n313 = Unbundle By Name(w576) -> ("Number Of Steps"=w573:u32)
            n314 = local read "hold steps"() -> (w572:i32)
            n315 = Add(x=w573, y=w572) -> (x+y=w571:u32)
            n316 = call "IVData.vi"("Action"=w574, "Array No."=u32 1 ("Action")) -> ("Array OUT"=w583:dbl[])  [unwired: 3 in, 1 out]
            n317 = Array Subset(array=w583, index=0, length=w571) -> (w580:dbl[])
            n318 = Absolute Value(x=w580) -> (abs(x)=w579:dbl[])
            n319 = case shown="\"microAmps\"" w581 {
              tunnel: [w586 w587 w591] -> w585
              tunnel: w579 -> [w586 w589 w592]
              frame .."nanoAmps" {
              }
              frame "microAmps" {
                n320 = Divide(x=w589, y=1000.0) -> (x/y=w587:dbl[])
              }
              frame "milliAmps".. {
                n321 = Divide(x=w592, y=1000000.0) -> (x/y=w591:dbl[])
              }
            }
            n322 = call "IVData.vi"("Action"=w574, "Array No."=u32 0 ("Action")) -> ("Array OUT"=w570:dbl[])  [unwired: 3 in, 1 out]
            n323 = Absolute Value(x=w570) -> (abs(x)=w569:dbl[])
            n324 = Bundle(w569, w585) -> (w582:cluster{dbl[], dbl[]})  [unwired: 1 in]
            n325 = local write "Igraph"(w582) -> ()
          }
        }
        n326 = Not Or(1:"quit (no save)", 2:"Quit & Save") -> (0:w563:bool)
      }
      n327 = global read "QC_MeasurementSetup.vi" "IV Measurement Parameters"() -> (w518:T7)
      n328 = Unbundle By Name(w518) -> ("Temperature Readout"=w517:enum16{"Read Arduino", "Enter manually"}, "Arduino"=w511:refnum<class "ArduinoControl.lvclass">)
      n329 = case shown="\"Read Arduino\"" w517 {
        tunnel: w511 -> [_ w559]
        frame "Enter manually", Default {
        }
        frame "Read Arduino" {
          n330 = call "ArduinoClose.vi"("ArduinoControl in"=w559) -> ()  [unwired: 9 in, 2 out]
        }
      }
      n331 = case shown="True" w521 {
        tunnel: [FALSE w603] -> w523
        frame False {
        }
        frame True {
          n332 = Two Button Dialog(message="Are you sure you don't want to save the data?", 1:"Quit" ("F button name (\"Cancel\")"), 2:"Save data" ("T button name (\"OK\")")) -> (T button?=w603:bool)
        }
      }
      n333 = Or(x=w522, y=w523) -> (x .or. y?=w516:bool)
      n334 = flat-sequence {
        tunnel: w516 -> [w524]
        tunnel: [w524] -> w512
        tunnel: [TRUE] -> w510
        frame #0 {
          n335 = global read "QC_MeasurementSetup.vi" "IV Measurement Parameters"() -> (w534:T7)
          n336 = Unbundle By Name(w534) -> ("V_breakdown Limit [V]"=w528:dbl, "Number Of Steps"=w529:u32)
          n337 = case shown="True" w524 {
            tunnel: ["" w558] -> w535
            tunnel: [_ w541] -> w533
            tunnel: w529 -> [_ w539]
            frame False {
            }
            frame True {
              w553 = T3."Read Array" ("Action")
              n338 = local read "hold steps"() -> (w538:i32)
              n339 = Add(x=w539, y=w538) -> (x+y=w537:u32)
              n340 = local write "STATUS 1"("Saving Data ...") -> ()
              n341 = call "IVData.vi"("Action"=w553, "Array No."=u32 3 ("Action")) -> ("Array OUT"=w555:dbl[])  [unwired: 3 in, 1 out]
              n342 = call "IVData.vi"("Action"=w553, "Array No."=u32 2 ("Action")) -> ("Array OUT"=w554:dbl[])  [unwired: 3 in, 1 out]
              n343 = call "IVData.vi"("Action"=w553, "Array No."=u32 0 ("Action")) -> ("Array OUT"=w548:dbl[])  [unwired: 3 in, 1 out]
              n344 = call "IVData.vi"("Action"=w553, "Array No."=u32 1 ("Action")) -> ("Array OUT"=w547:dbl[])  [unwired: 3 in, 1 out]
              n345 = call <vilib>:"Std Deviation and Variance.vi"("X"=w555) -> ("mean"=w542:dbl)  [unwired: 1 in, 2 out]
              n346 = call <vilib>:"Std Deviation and Variance.vi"("X"=w554) -> ("mean"=w543:dbl)  [unwired: 1 in, 2 out]
              n347 = Build Array(w548, w547) -> (w546:dbl[][])
              n348 = Transpose 2D Array(2D array=w546) -> (transposed array=w545:dbl[][])
              n349 = call "SaveDataFile.vi"("Arrays format"="%010.2f", "Humidity"=w542, "Array Titles"="Voltage[V] Current[nA]", "Temperature"=w543, "Actual array lengths"=w537, "no. of arrays"=2, "Data Array"=w545) -> ("Error Out"=w541:errorcluster, "Path + Filename OUT"=w558:string)  [unwired: 1 in, 2 out]
            }
          }
          n350 = Absolute Value(x=w528) -> (abs(x)=w527:dbl)
          n351 = call "ScanFeedback.vi"("measurement type"=T2."IV") -> ("V breakdown"=w526:dbl)  [unwired: 3 in, 5 out]
          n352 = Absolute Value(x=w526) -> (abs(x)=w525:dbl)
          n353 = Greater Or Equal?(x=w525, y=w527) -> (x >= y?=w530:bool)
          n354 = call "WriteLogFile.vi"("Data File"=w535, "Error In"=w533, "DUT passed?"=w530, "Value TechSpec criteria"=w526, "Files saved?"=w524) -> ()  [unwired: 6 in, 1 out]
        }
      }
      n355 = Select(t="Run finished.\nData saved." ("STATUS 1"), s=w512, f="Run finished.\nData not saved." ("STATUS 1")) -> (s? t:f=w515:string)
      n356 = local write "STATUS 1"(w515) -> ()
      "Done!" <- w510
    }
  }
